vi "Plotter_Queues_FGV.vi"(8 "error in (no error)":errorcluster, 11 "Initialize ?":bool) -> (0 "error out":errorcluster, 3 "Queues":T1)   [LabVIEW 2017]
uses:
  Controls/Plotter_Queues.ctl
  Controls/Plotter_Queue_Command_and_Data.ctl
  Controls/Plotter_Commands.ctl
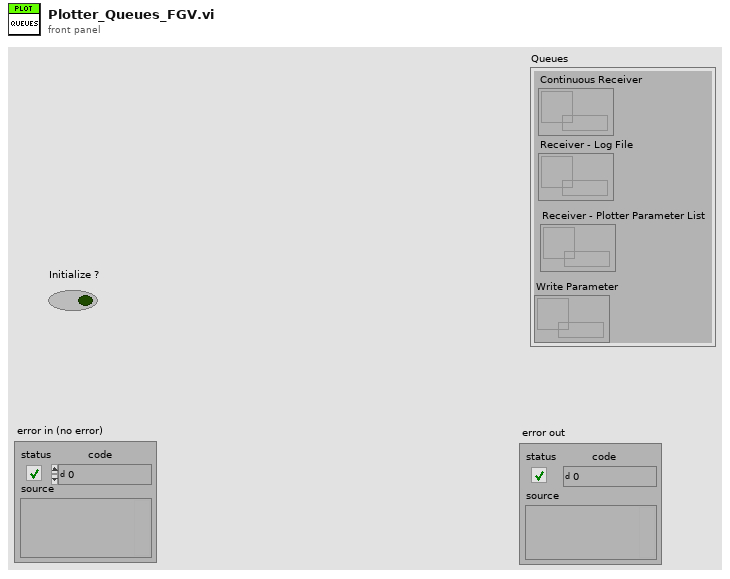
[diagram p1: front panel]
types:
  T1 = typedef "Plotter_Queues.ctl" = cluster{"Continuous Receiver":refnum<queue>, "Receiver - Log File":refnum<queue>, "Receiver - Plotter Parameter List":refnum<queue>, "Write Parameter":refnum<queue>}
  T2 = typedef "Plotter_Queue_Command_and_Data.ctl" = cluster{"Commands":T3, "Data":variant}
  T3 = typedef "Plotter_Commands.ctl" = enum16{"Idle", "Cont_RX_Open_Node", "Cont_RX_Flush_Serial_Port", "Cont_Rx_Log_Write", "Plot_Update", "Exit"}
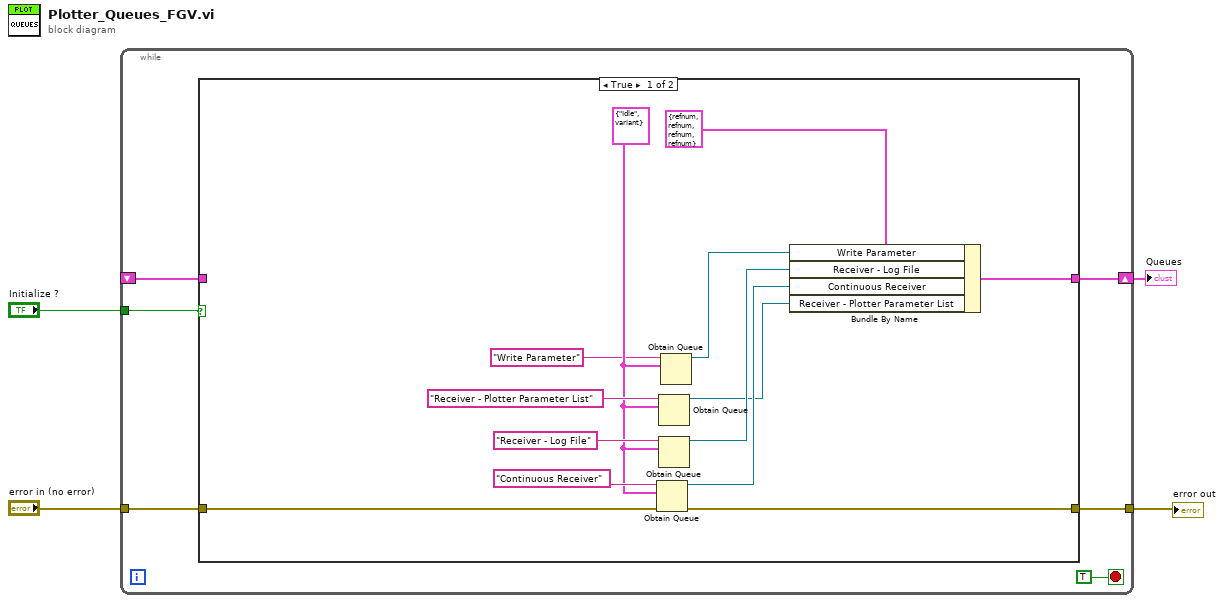
[diagram p0: block diagram]
diagram:
  n1 = while {
    tunnel: "error in (no error)" -> [w9]
    tunnel: "Initialize ?" -> [w8]
    tunnel: [w7] -> w2
    shift-right: [w6] -> w1
    shift-left: _ -> [w5]
    stop <- TRUE stop-if-true
    n2 = case shown="True" w8 {
      tunnel: w9 -> [w23 w24]
      tunnel: [w22 w24] -> w7
      tunnel: [w16 w25] -> w6
      tunnel: w5 -> [_ w25]
      frame True {
        w13 = T2 {"Commands"=enum."Idle", "Data"=variant} ("Plotter_Queue_Command_and_Data")
        n3 = Obtain Queue(name (unnamed)="Continuous Receiver", element data type=w13, error in (no error)=w23) -> (queue out=w17:refnum<queue>, error out=w22:errorcluster)  [unwired: 2 in, 1 out]
        n4 = Obtain Queue(name (unnamed)="Receiver - Plotter Parameter List", element data type=w13) -> (queue out=w14:refnum<queue>)  [unwired: 3 in, 2 out]
        n5 = Obtain Queue(name (unnamed)="Receiver - Log File", element data type=w13) -> (queue out=w18:refnum<queue>)  [unwired: 3 in, 2 out]
        n6 = Obtain Queue(name (unnamed)="Write Parameter", element data type=w13) -> (queue out=w11:refnum<queue>)  [unwired: 3 in, 2 out]
        n7 = Bundle By Name(cluster=T1 {"Continuous Receiver"=refnum, "Receiver - Log File"=refnum, "Receiver - Plotter Parameter List"=refnum, "Write Parameter"=refnum}, "Write Parameter"=w11, "Receiver - Log File"=w18, "Continuous Receiver"=w17, "Receiver - Plotter Parameter List"=w14) -> (w16:T1)
      }
      frame False {
      }
    }
  }
  "error out" <- w2
  "Queues" <- w1
